vi "JSONRPC-InvokeMethod.vi"(6 "variableArray":string[][](array[string]), 7 "method":T1(ring), 8 "error in (no error)":errorcluster, 11 "params":string[](array[string])) -> (0 "error out":errorcluster, 2 "resultper":string, 3 "result":string)   [LabVIEW 2020]
doc: "Invokes the actual implementation of a RIP <b>method</b>."
uses:
  Configuration/Global_Configurations.vi
  JSONRPC-GetAsString.vi
  JSONRPC-ArrayToString_Cluster.vi
  JSONRPC-ArrayToString_String.vi
  JSONRPC-GetAsArray.vi
panel:
  # "InvokeMethod"
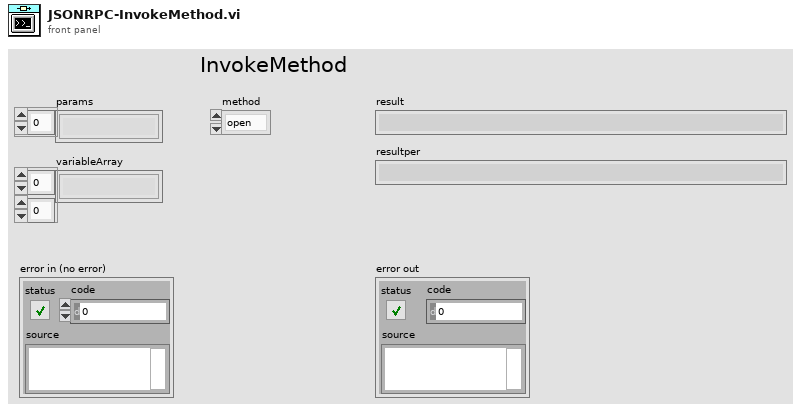
[diagram p1: front panel]
types:
  T1 = enum16{"open", "close", "start", "stop", "get", "set", "info", "UNDEFINED"}
  T2 = enum16{"Parse error", "Invalid request", "Method not found", "Invalid params", "Internal error", "Server error", ""}
  T3 = cluster{"Path":path, "Name":string, "Authors":string, "Keywords":string, "Description":string, "Cameras":cluster{"Base URL":string, "Path":string, "Name":string}[], "Sampling":cluster{"Sampled Variable":string, "Delta":dbl}[], "Sampling Freq":u32}[]
  T4 = cluster{"Name":string, "Type":string, "Min":string, "Max":string, "Precision":string, "Description":string}[]
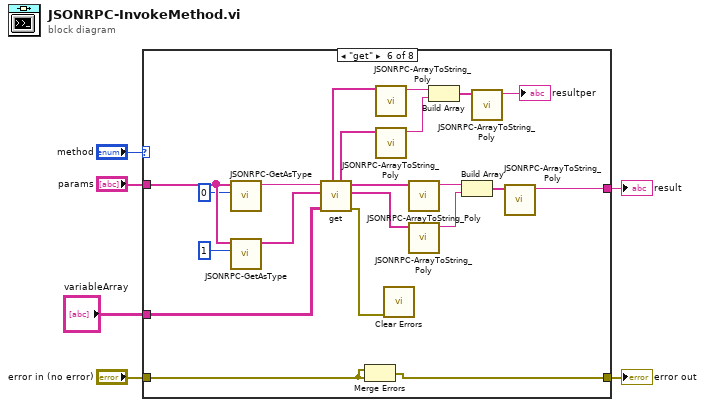
[diagram p0: block diagram]
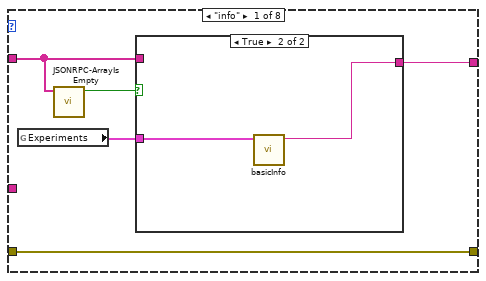
[diagram p2: hidden frame]
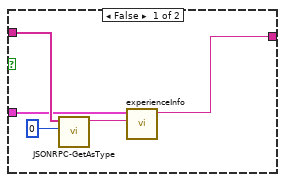
[diagram p3: hidden frame]
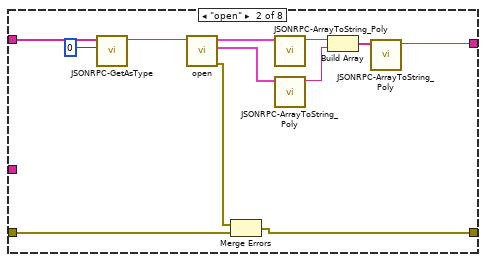
[diagram p4: hidden frame]
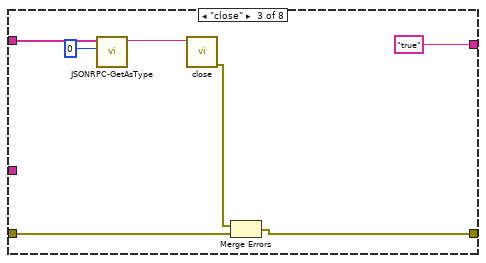
[diagram p5: hidden frame]
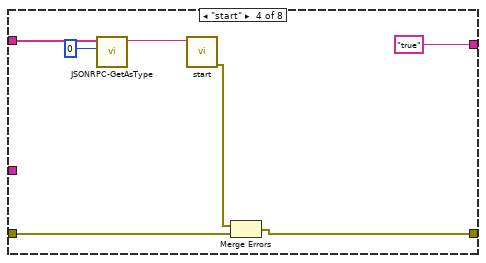
[diagram p6: hidden frame]
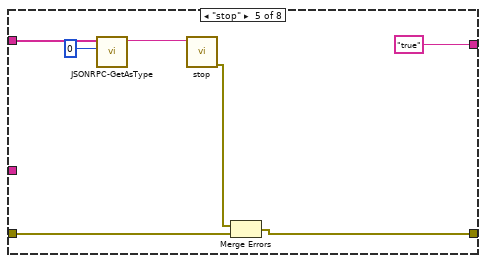
[diagram p7: hidden frame]
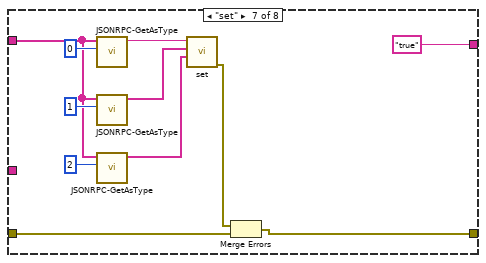
[diagram p8: hidden frame]
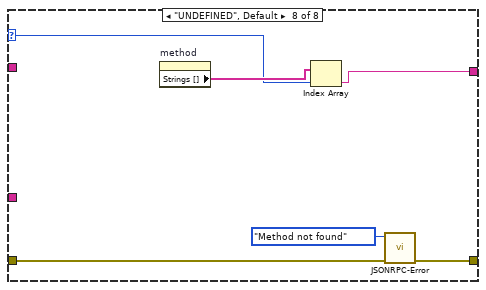
[diagram p9: hidden frame]
diagram:
  n1 = case shown="\"get\"" "method" {
    selector: "method" -> [_ _ _ _ _ _ _ w85]
    tunnel: "params" -> [w10 w23 w32 w39 w48 w66 w75 _]
    tunnel: [w11 w29 w35 w42 w49 w72 w81 w88] -> w4
    tunnel: "error in (no error)" -> [w11 w30 w36 w43 w50 w61 w82 w87]
    tunnel: [w8 w19 "true" "true" "true" w59 "true" w84] -> w2
    tunnel: "variableArray" -> [_ _ _ _ _ w58 _ _]
    frame "info" {
      n2 = global read "Global_Configurations.vi" "Experiments"() -> (w7:T3)
      n3 = call "JSONRPC-ArrayIsEmpty.vi"("input array"=w10) -> ("empty?"=w9:bool)  [unwired: 10 in]
      n4 = case shown="True" w9 {
        tunnel: w10 -> [w13 _]
        tunnel: [w16 w18] -> w8
        tunnel: w7 -> [w12 w17]
        frame False {
          n5 = call-poly "JSONRPC-GetAsType.vi"("index"=0, "params"=w13) -> ("output"=w14:string)  [unwired: 9 in]
          n6 = call "experienceInfo.vi"("info in"=w14, "Experiments"=w12) -> ("info out"=w16:string)  [unwired: 9 in]
        }
        frame True {
          n7 = call "basicInfo.vi"("Experiments"=w17) -> ("String"=w18:string)  [unwired: 10 in]
        }
      }
    }
    frame "open" {
      n8 = call-poly "JSONRPC-GetAsType.vi"("index"=0, "params"=w23) -> ("output"=w24:string)  [unwired: 9 in]
      n9 = call "open.vi"("Experience ID"=w24) -> ("error out"=w28:errorcluster, "Indicators_list"=w20:T4, "Controls_list"=w21:T4)  [unwired: 8 in]
      n10 = Merge Errors(w28, w30) -> (w29:errorcluster)
      n11 = call-poly "JSONRPC-ArrayToString_Poly.vi"("List"=w21) -> ("Output"=w22:string)  [unwired: 10 in]
      n12 = call-poly "JSONRPC-ArrayToString_Poly.vi"("List"=w20) -> ("Output"=w27:string)  [unwired: 10 in]
      n13 = Build Array(w22, w27) -> (w26:string[])
      n14 = call-poly "JSONRPC-ArrayToString_Poly.vi"("Array"=w26) -> ("Output"=w19:string)  [unwired: 10 in]
    }
    frame "close" {
      n15 = call-poly "JSONRPC-GetAsType.vi"("index"=0, "params"=w32) -> ("output"=w33:string)  [unwired: 9 in]
      n16 = call "close.vi"("Experience ID"=w33) -> ("error out"=w37:errorcluster)  [unwired: 10 in]
      n17 = Merge Errors(w37, w36) -> (w35:errorcluster)
    }
    frame "start" {
      n18 = call-poly "JSONRPC-GetAsType.vi"("index"=0, "params"=w39) -> ("output"=w40:string)  [unwired: 9 in]
      n19 = call "start.vi"("Experience ID"=w40) -> ("error out"=w44:errorcluster)  [unwired: 10 in]
      n20 = Merge Errors(w44, w43) -> (w42:errorcluster)
    }
    frame "stop" {
      n21 = call-poly "JSONRPC-GetAsType.vi"("index"=0, "params"=w48) -> ("output"=w46:string)  [unwired: 9 in]
      n22 = call "stop.vi"("Experience ID"=w46) -> ("error out"=w51:errorcluster)  [unwired: 10 in]
      n23 = Merge Errors(w51, w50) -> (w49:errorcluster)
    }
    frame "get" {
      n24 = call-poly "JSONRPC-GetAsType.vi"("index"=0, "params"=w66) -> ("output"=w62:string)  [unwired: 9 in]
      n25 = call-poly "JSONRPC-GetAsType.vi"("index"=1, "params"=w66) -> ("output"=w63:string[])  [unwired: 9 in]
      n26 = call "get.vi"("variableArray"=w58, "variables"=w63, "Experience ID"=w62) -> ("error out"=w60:errorcluster, "values"=w70:string[], "names"=w68:string[], "values 2"=w55:string[], "names 2"=w54:string[])  [unwired: 4 in]
      n27 = Merge Errors(w61, w61) -> (w72:errorcluster)
      n28 = call-poly "JSONRPC-ArrayToString_Poly.vi"("Array"=w54) -> ("Output"=w56:string)  [unwired: 10 in]
      n29 = call-poly "JSONRPC-ArrayToString_Poly.vi"("Array"=w55) -> ("Output"=w53:string)  [unwired: 10 in]
      n30 = call <vilib>:"Clear Errors.vi"("error in (no error)"=w60) -> ()  [unwired: 5 in, 2 out]
      n31 = call-poly "JSONRPC-ArrayToString_Poly.vi"("Array"=w68) -> ("Output"=w67:string)  [unwired: 10 in]
      n32 = call-poly "JSONRPC-ArrayToString_Poly.vi"("Array"=w70) -> ("Output"=w71:string)  [unwired: 10 in]
      n33 = Build Array(w56, w53) -> (w57:string[])
      n34 = Build Array(w67, w71) -> (w69:string[])
      n35 = call-poly "JSONRPC-ArrayToString_Poly.vi"("Array"=w57) -> ("Output"=→"resultper":string)  [unwired: 10 in]
      n36 = call-poly "JSONRPC-ArrayToString_Poly.vi"("Array"=w69) -> ("Output"=w59:string)  [unwired: 10 in]
    }
    frame "set" {
      n37 = call-poly "JSONRPC-GetAsType.vi"("index"=0, "params"=w75) -> ("output"=w80:string)  [unwired: 9 in]
      n38 = call-poly "JSONRPC-GetAsType.vi"("index"=1, "params"=w75) -> ("output"=w78:string[])  [unwired: 9 in]
      n39 = call-poly "JSONRPC-GetAsType.vi"("index"=2, "params"=w75) -> ("output"=w74:string[])  [unwired: 9 in]
      n40 = call "set.vi"("values"=w74, "variables"=w78, "Experience ID"=w80) -> ("error out"=w83:errorcluster)  [unwired: 8 in]
      n41 = Merge Errors(w83, w82) -> (w81:errorcluster)
    }
    frame "UNDEFINED", Default {
      n42 = property on="method" class="Enum (strict)"() -> ("Strings []"=w86:string[])  [unwired: 2 in, 2 out]
      n43 = Index Array(array=w86, index=w85) -> (element=w84:string)
      n44 = call "JSONRPC-Error.vi"("error in"=w87, "Type"=T2."Method not found") -> ("error out"=w88:errorcluster)  [unwired: 9 in]
    }
  }
  "error out" <- w4
  "result" <- w2
